vi "DDS9959 Ramp String.vi"(2 "Clock Frequency (MHz)":dbl, 3 "Ramp Step (us)":dbl max=1.0) -> (1 "String":string)   [LabVIEW 2012]
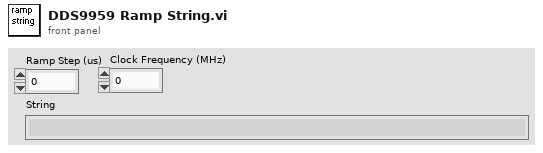
[diagram p1: front panel]
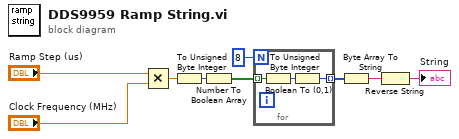
[diagram p0: block diagram]
diagram:
  n1 = Multiply(x="Ramp Step (us)", y="Clock Frequency (MHz)") -> (x*y=w4:dbl)
  n2 = To Unsigned Byte Integer(number=w4) -> (unsigned 8bit integer=w3:u8)
  n3 = Number To Boolean Array(number=w3) -> (Boolean array=w5:bool[])
  n4 = for {
    N: 8 -> [_]
    tunnel: w5 -> [w12] mode=indexing
    tunnel: [w10] -> w9 mode=indexing
    n5 = Boolean To (0,1)(Boolean=w12) -> (0, 1=w11:i16)
    n6 = To Unsigned Byte Integer(number=w11) -> (unsigned 8bit integer=w10:u8)
  }
  n7 = Byte Array To String(unsigned byte array=w9) -> (string=w8:string)
  n8 = Reverse String(1:w8) -> (0:→"String":string)
